vi "uNotify Optimize.vi"(8 "error in (no error)":errorcluster, 10 "Listener Transport in":refnum<class "uTransport.lvclass">, 11 "uNotifyMode in":refnum<class "uNotifyMode.lvclass">) -> (0 "error out":errorcluster, 2 "Listener Transport out":refnum<class "uTransport.lvclass">, 3 "uNotifyMode out":refnum<class "uNotifyMode.lvclass">)   [LabVIEW 2023, in "uLib.lvlib" / "uNotifyMode.lvclass"]
doc: "Call this VI to force the object to optimize its execution for the type of the listener transport; in order to improve the data throughput."
uses:
  uNotifyMode.lvclass
  uTransport/uTransport/uTransport.lvclass
  uActor/uActor/uActor.lvclass
  uActor/uActor/uActor.lvclass/uActor.ctl
  uNotifyMode.lvclass/uNotifyMode.ctl
  uActor/uActor/uActor_Get Self Transport.vi
  uTransport/uTransport_uActor/uTransport_uActor.lvclass
  U:/Projects/uLib/Src/uFramework/uTransport/uTransport.lvclass
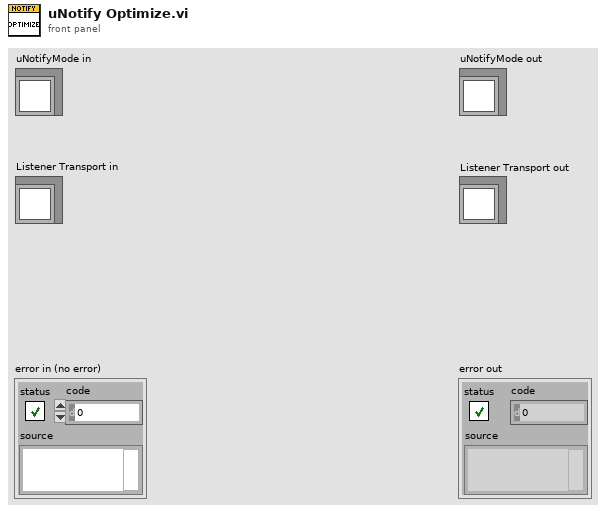
[diagram p1: front panel]
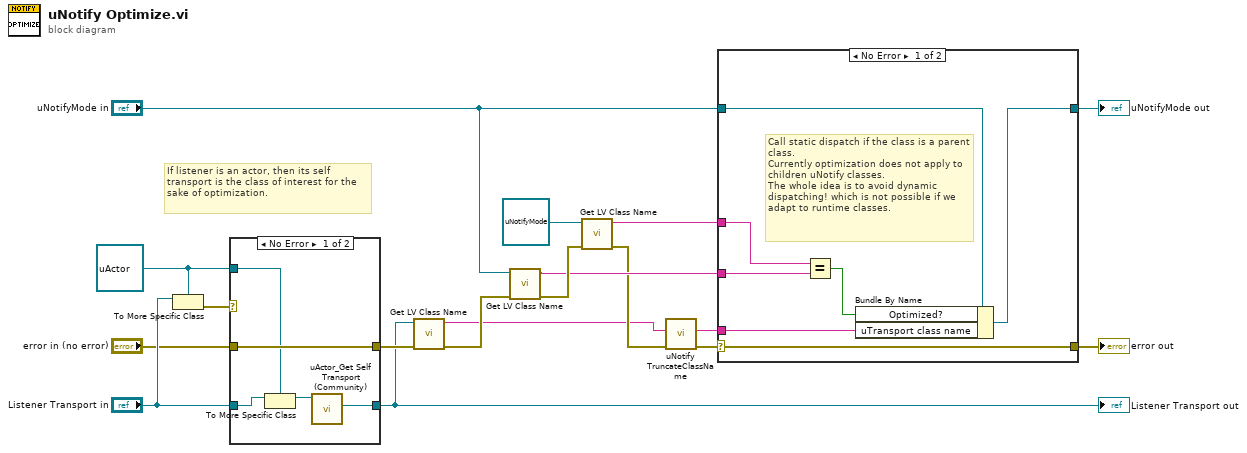
[diagram p0: block diagram]
diagram:
  w1 = refnum<class "uActor.lvclass"> refnum ("uFramework.lvlib:uActor.lvclass")
  # "If listener is an actor, then its self transport is the class of interest for the sake of optimization."
  n1 = To More Specific Class(target class=w1, reference="Listener Transport in") -> (error out=w8:errorcluster)  [unwired: 1 in, 1 out]
  n2 = case shown="No Error" w8 {
    tunnel: "Listener Transport in" -> [w22 w24]
    tunnel: "error in (no error)" -> [w23 w25]
    tunnel: [w23 w25] -> w5
    tunnel: [w19 w24] -> w2
    tunnel: w1 -> [w21 _]
    frame No Error {
      n3 = To More Specific Class(target class=w21, reference=w22) -> (specific class reference=w20:refnum<class "uActor.lvclass">)  [unwired: 1 in, 1 out]
      n4 = call "uActor_Get Self Transport (Community).vi"("uActor in"=w20) -> ("Actor Transport"=w19:refnum<class "uTransport_uActor.lvclass">)  [unwired: 9 in, 1 out]
    }
    frame Error {
    }
  }
  "Listener Transport out" <- w2
  n5 = call <vilib>:"Get LV Class Name.vi"("error in (no error)"=w5, "object"=w2) -> ("error out"=w4:errorcluster, "class name"=w3:string)  [unwired: 8 in]
  n6 = call <vilib>:"Get LV Class Name.vi"("error in (no error)"=w4, "object"="uNotifyMode in") -> ("error out"=w15:errorcluster, "class name"=w13:string)  [unwired: 8 in]
  n7 = call <vilib>:"Get LV Class Name.vi"("error in (no error)"=w15, "object"=refnum<class "uNotifyMode.lvclass"> refnum ("uBroker.lvlib:uNotifyMode.lvclass")) -> ("error out"=w11:errorcluster, "class name"=w12:string)  [unwired: 8 in]
  n8 = call "uNotify TruncateClassName.vi"("error in (no error)"=w11, "LV Class Name in"=w3) -> ("error out"=w10:errorcluster, "LV Class Name out"=w9:string)  [unwired: 8 in]
  n9 = case shown="No Error" w10 {
    selector: w10 -> [w32 w34]
    tunnel: [w32 w34] -> w18
    tunnel: [w30 w33] -> w17
    tunnel: "uNotifyMode in" -> [w29 w33]
    tunnel: w9 -> [w31 _]
    tunnel: w13 -> [w28 _]
    tunnel: w12 -> [w27 _]
    frame No Error {
      # "Call static dispatch if the class is a parent class.\nCurrently optimization does not apply to children uNotify classes.\nThe whole idea is to avoid dynamic dispatching! which is not possible if we adapt to runtime classes."
      n10 = Equal?(x=w27, y=w28) -> (x = y?=w26:bool)
      n11 = Bundle By Name(cluster=w29, "Optimized?"=w26, "uTransport class name"=w31) -> (w30:refnum<class "uNotifyMode.lvclass">)
    }
    frame Error {
    }
  }
  "error out" <- w18
  "uNotifyMode out" <- w17
